vi "Launch Controller.vi"(8 "error in":errorcluster) -> ()   [LabVIEW 2015]
doc: "This VI executes continuously carrying out the current operation and responding to updates or new operations. It will often contain the timing or control code that is difficult to place directly in TeleOp. This VI generally opens all sensors and motors and isolates the rest of the robot code from knowing how the operations are carried out."
uses:
  Launch Operations.ctl
  Launch Setpoints.ctl
  <vilib>/Rock Robotics/WPI/SafetyOutput/WPI_SafetyOutputConfigMenu.ctl
  <vilib>/Rock Robotics/SystemInterfaces/DIO/FPGA_DIOPWMChannel.ctl
  <vilib>/addons/control/pid/NI_PID_pid.lvlib
  <vilib>/addons/control/pid/pid.llb/PID (DBL).vi
  <vilib>/Rock Robotics/WPI/MotorControl/WPI_MotorControlOpen SPARK.vi
  <vilib>/Rock Robotics/Network Tables/NT Write Boolean.vi
panel:
  in  "PID gains (flywheel R speed)":T1={"proportional gain (Kc)"=0.6, "integral time (Ti, min)"=0.01, "derivative time (Td, min)"=0.0}
  in  "Angle Tolerance":dbl=0.05 format="%#_13g"
  in  "PID gains (launcher angle set)":T1={"proportional gain (Kc)"=0.6, "integral time (Ti, min)"=0.01, "derivative time (Td, min)"=0.0}
  in  "PID gains (flywheel L speed)":T1={"proportional gain (Kc)"=0.6, "integral time (Ti, min)"=0.01, "derivative time (Td, min)"=0.0}
  out "Current\nCmd":string
  # "Tip: It may be helpful to observe inputs and sensor values.\nYou may also want to display tuning or debugging controls."
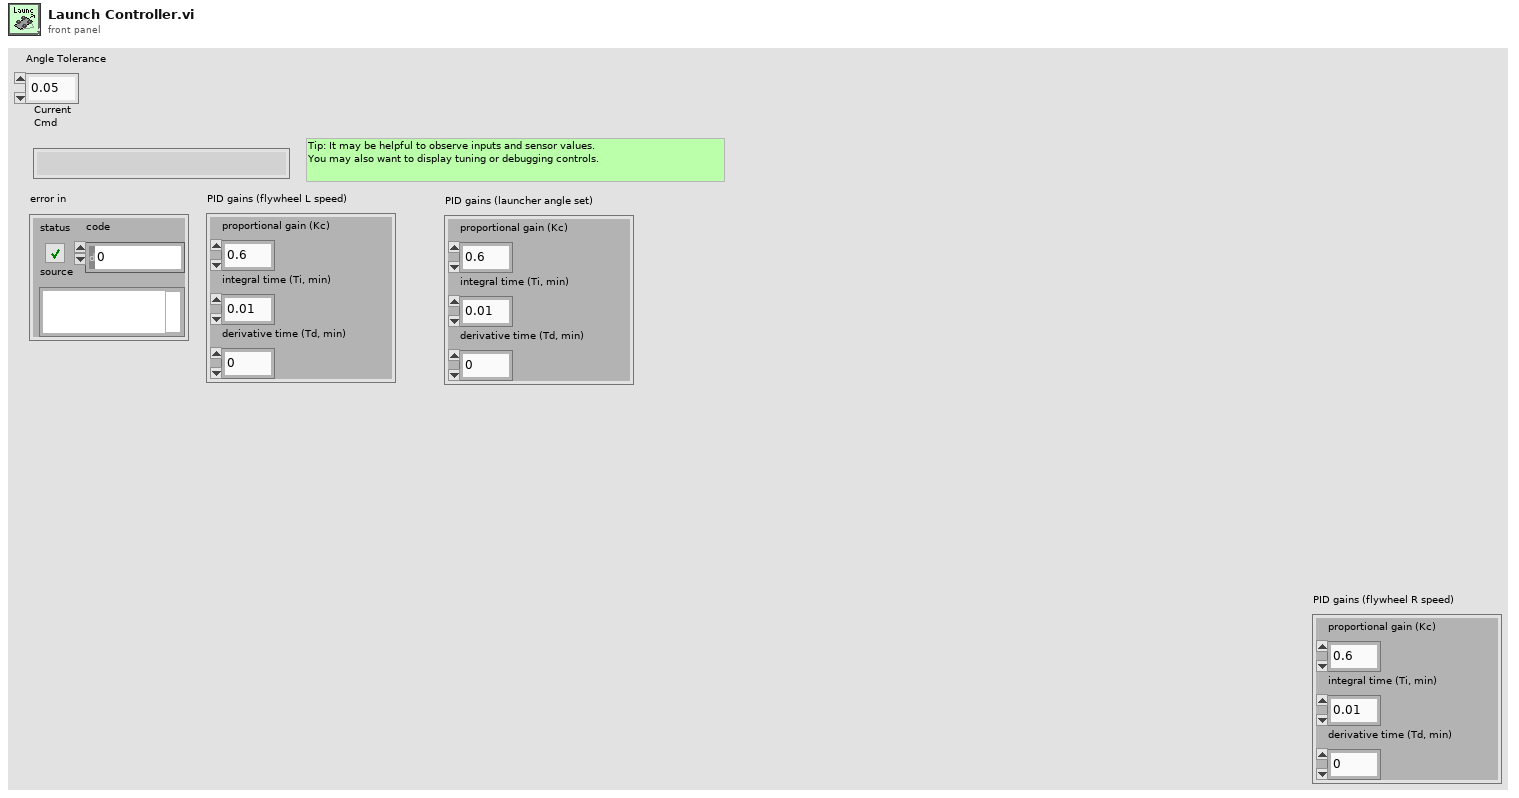
[diagram p1: front panel]
types:
  T1 = cluster{"proportional gain (Kc)":dbl, "integral time (Ti, min)":dbl, "derivative time (Td, min)":dbl}
  T2 = typedef "WPI_SafetyOutputConfigMenu.ctl" = enum16{"Enable", "Disable"}
  T3 = typedef "FPGA_DIOPWMChannel.ctl" = enum8{"PWM 0", "PWM 1", "PWM 2", "PWM 3", "PWM 4", "PWM 5", "PWM 6", "PWM 7", "PWM 8", "PWM 9", "PWM MXP 0", "PWM MXP 1", "PWM MXP 2", "PWM MXP 3", "PWM MXP 4", "PWM MXP 5", "PWM MXP 6", "PWM MXP 7", "PWM MXP 8", "PWM MXP 9", "Invalid"}
  T4 = typedef "Launch Setpoints.ctl" = cluster{"Operation":T5, "Setpoint":dbl, "Duration":dbl}
  T5 = typedef "Launch Operations.ctl" = enum16{"Reserve", "Read Current", "Immediate", "Zero", "Launcher Test", "Set Velocity", "Set Angle", "Manual Angle Test"}
  T6 = typedef "WPI_MotorControlDeviceRef.ctl" = cluster{"DeviceStatus":errorcluster, "Type":T7, "PWM":cluster{"PWM Channel":T3, "DeadBand":T8}, "CAN":cluster{"Device Number":u8, "Control Mode":T9, "Semaphore":T10, "Max Vout":dbl, "TalonSRX Control Mode":T11}, "Invert":bool}
  T7 = typedef "WPI_MotorControlType.ctl" = enum16{"PWM", "CAN", "CANTalonSRX"}
  T8 = typedef "WPI_PWMDeadband.ctl" = cluster{"Name":string, "maxPositivePwm":i32, "minPositivePwm":i32, "centerPwm":i32, "maxNegativePwm":i32, "minNegativePwm":i32, "angularRange":u16}
  T9 = typedef "WPI_CANJaguar_ControlMode.ctl" = enum8{"Percent VBus", "Current", "Speed", "Position", "Voltage"}
  T10 = typedef "Semaphore RefNum" = refnum<k1>
  T11 = typedef "WPI_CANTalonSRX_APIControlMode.ctl" = enum8{"Percent VBus", "Speed", "Position", "Slave", "Unchanged / Invalid", "Voltage Compensation", "Current", "Motion Profile"}
  T12 = typedef "WPI_SwitchDevRef.ctl" = cluster{"DevStatus":errorcluster, "DIO Channel":T13, "CntIndex":T14, "Normally Closed":bool}
  T13 = typedef "FPGA_DIOChannel.ctl" = enum8{"DIO 0", "DIO 1", "DIO 2", "DIO 3", "DIO 4", "DIO 5", "DIO 6", "DIO 7", "DIO 8", "DIO 9", "DIO MXP 0", "DIO MXP 1", "DIO MXP 2", "DIO MXP 3", "DIO MXP 4", "DIO MXP 5", "DIO MXP 6", "DIO MXP 7", "DIO MXP 8", "DIO MXP 9", "DIO MXP 10", "DIO MXP 11", "DIO MXP 12", "DIO MXP 13", "DIO MXP 14", "DIO MXP 15", "Invalid"}
  T14 = typedef "FPGA_CounterCtrSystemIndex.ctl" = enum8{"Ctr 0", "Ctr 1", "Ctr 2", "Ctr 3", "Ctr 4", "Ctr 5", "Ctr 6", "Ctr 7", "Invalid"}
  T15 = typedef "WPI_EncoderDevRef.ctl" = cluster{"DevStatus":errorcluster, "EncoderIndex":T16, "CounterIndex":T14, "DistancePerCount":dbl, "Decoding Type":T17}
  T16 = typedef "FPGA_EncoderIdx.ctl" = enum8{"Enc 0", "Enc 1", "Enc 2", "Enc 3", "Enc 4", "Enc 5", "Enc 6", "Enc 7", "Invalid"}
  T17 = typedef "WPI_EncoderType.ctl" = enum16{"1x", "2x", "4x"}
  T18 = typedef "Command Status Info.ctl" = cluster{"Name":string, "Status":T19, "notifier out":T20}
  T19 = typedef "Completion Status.ctl" = enum16{"Successful", "Aborted", "Incomplete"}
  T20 = typedef "Completion Notifier.ctl" = refnum<notifier>
  T21 = cluster{"Default Command":T4, "Command Timing":cluster{"Start Time (ms)":u32, "Iterations":i32}, "Command Arguments":cluster{"Command Info":T18, "Description":string, "Default Command":T4, "notifier out":refnum<notifier>, "Subsystem Name":string}}
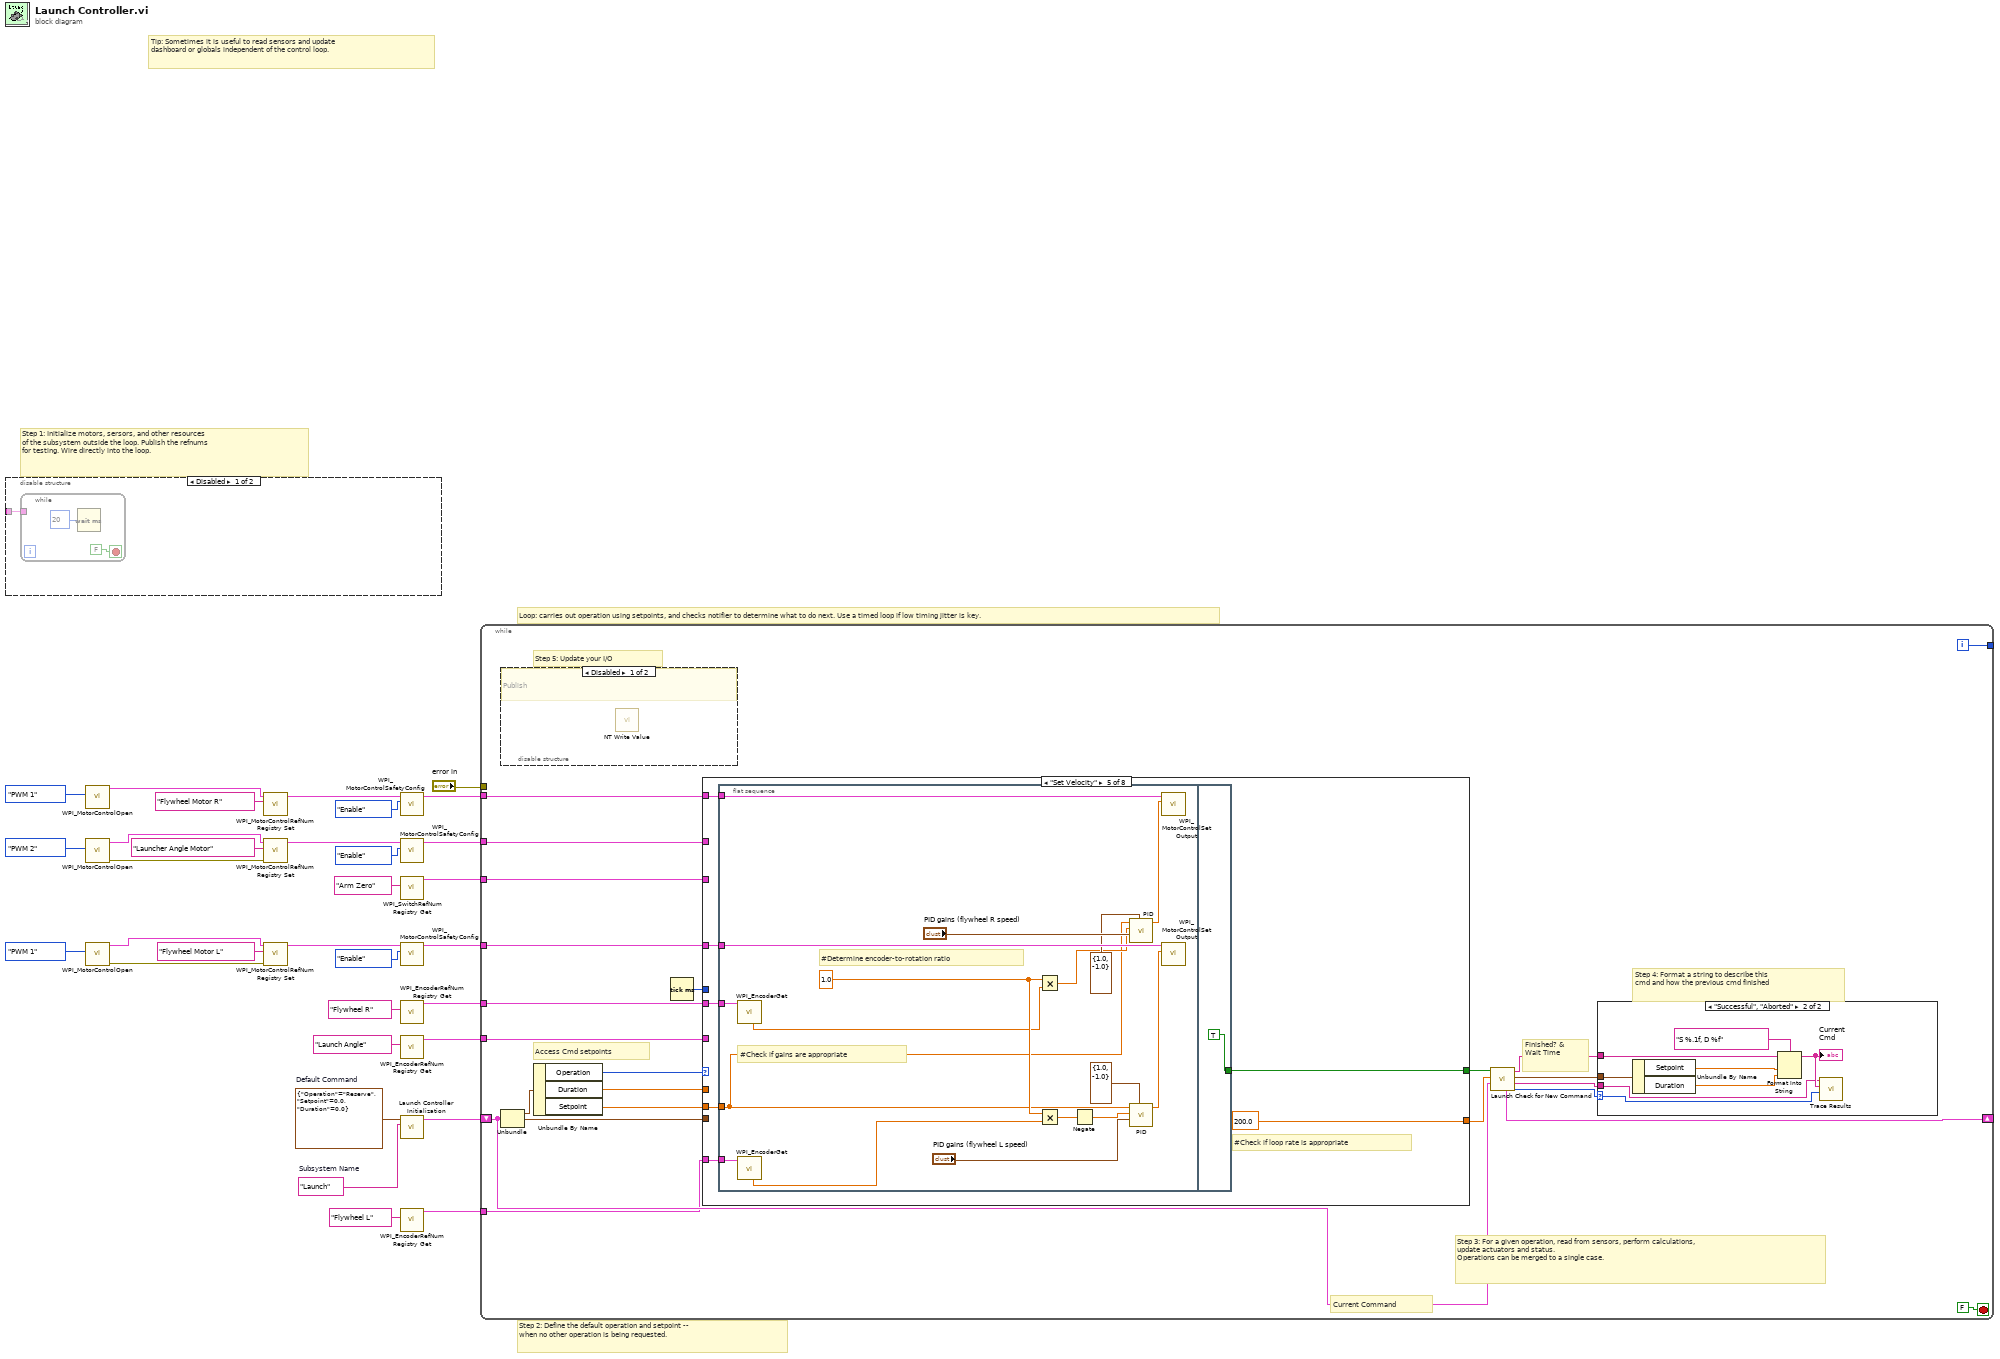
[diagram p0: block diagram]
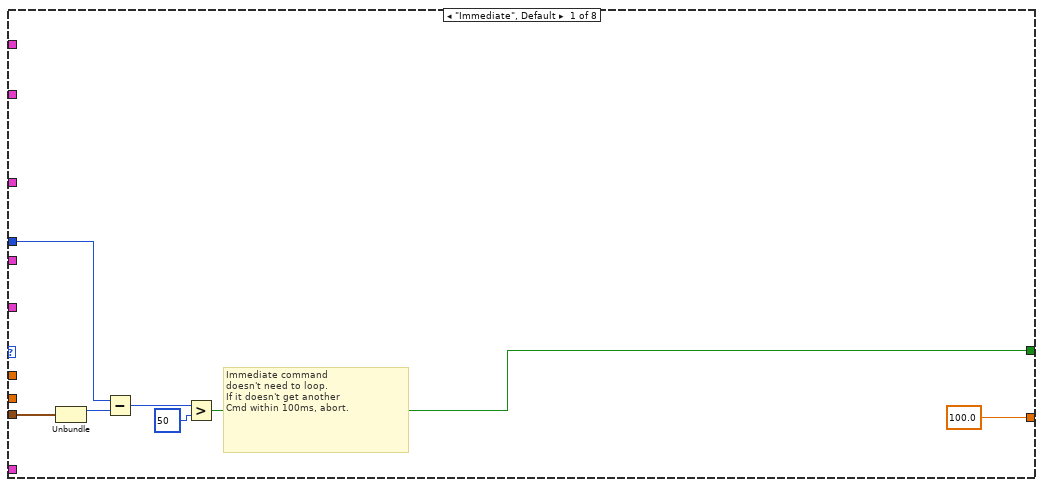
[diagram p5: hidden frame]
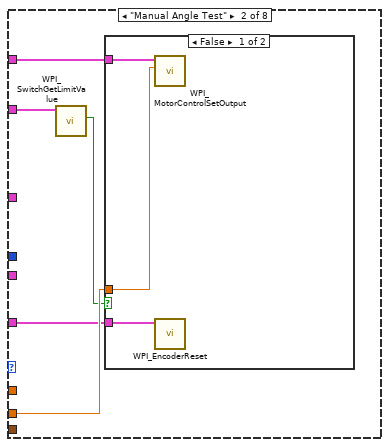
[diagram p6: hidden frame]
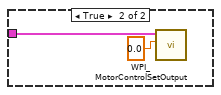
[diagram p7: hidden frame]
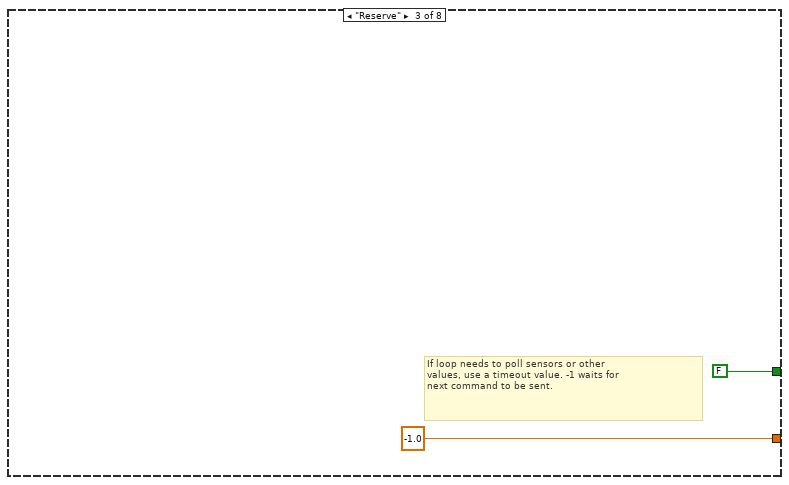
[diagram p8: hidden frame]
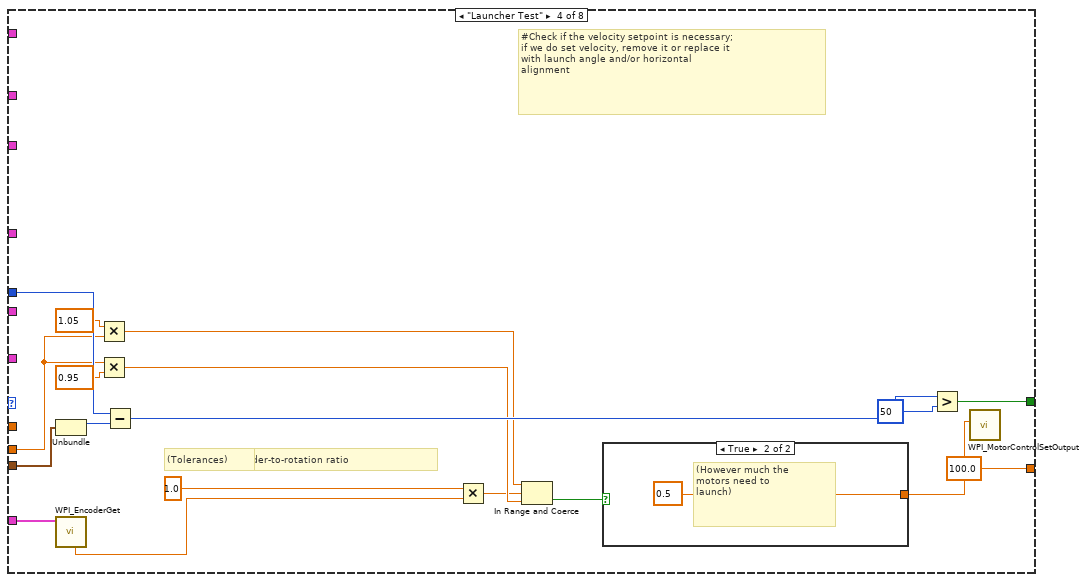
[diagram p9: hidden frame]
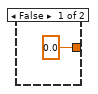
[diagram p10: hidden frame]
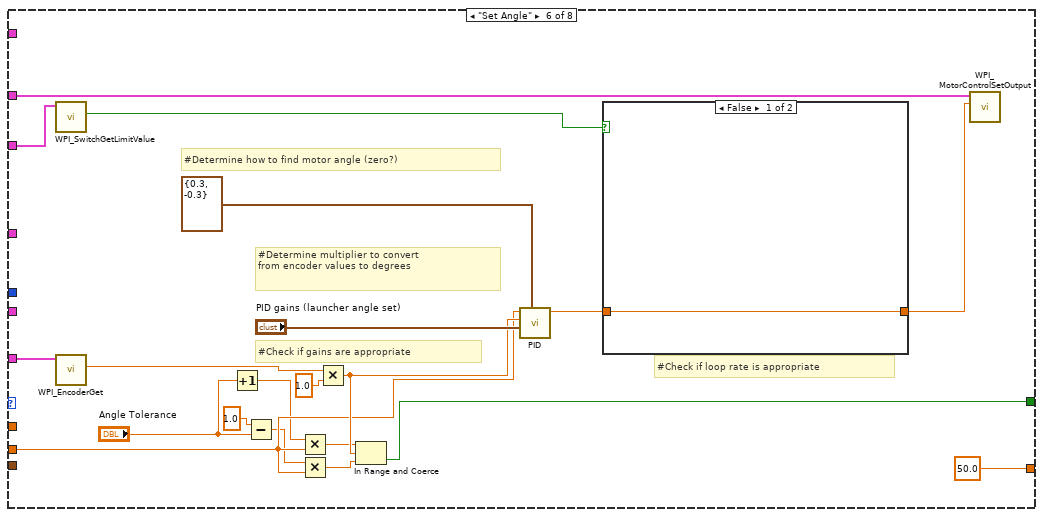
[diagram p11: hidden frame]
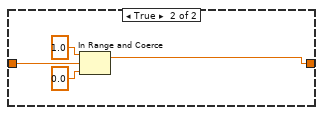
[diagram p12: hidden frame]
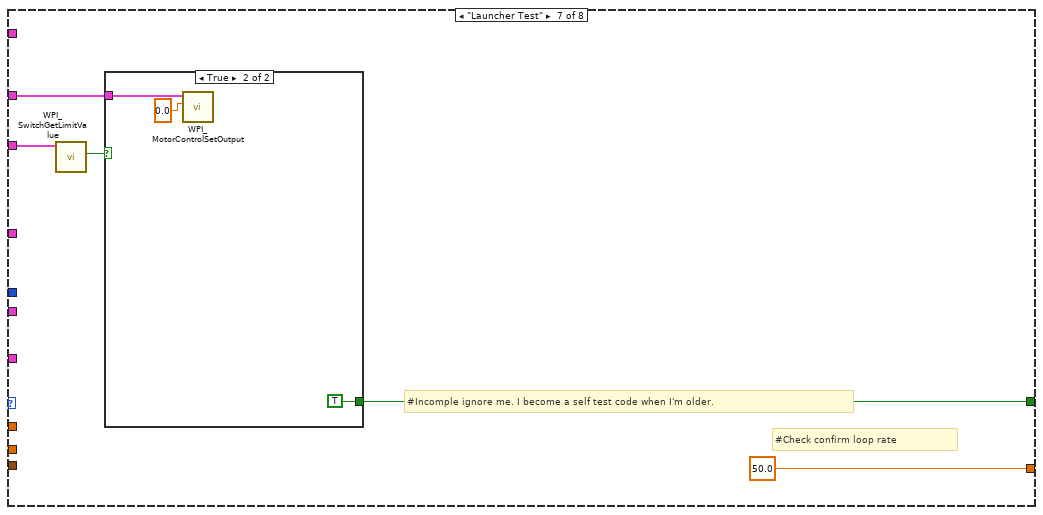
[diagram p13: hidden frame]
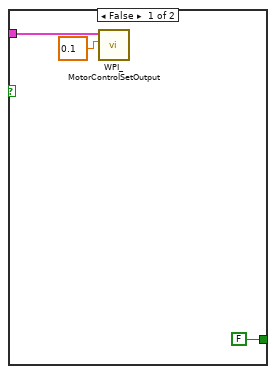
[diagram p14: hidden frame]
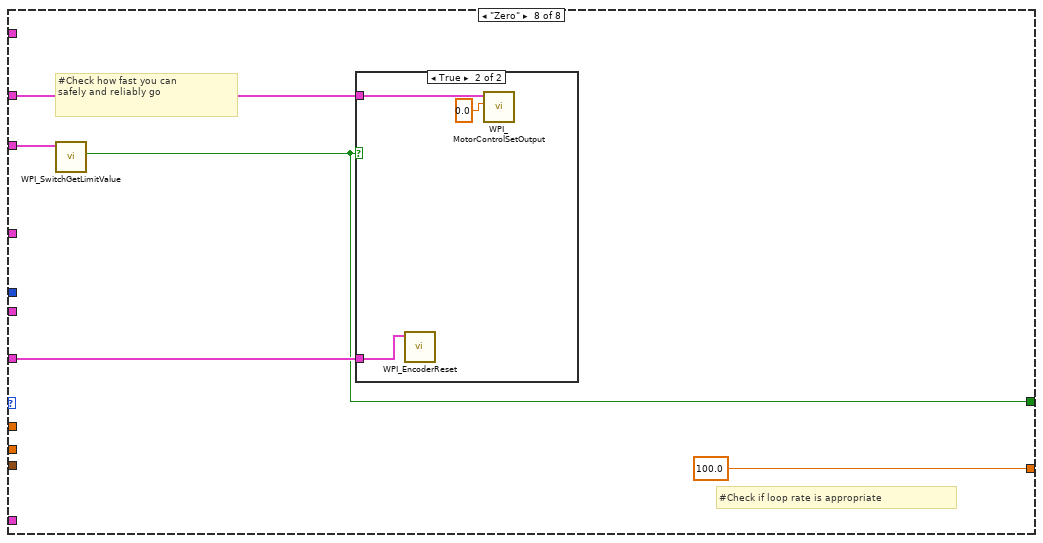
[diagram p15: hidden frame]
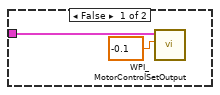
[diagram p16: hidden frame]
diagram:
  w29 = T4 {"Operation"=enum."Reserve", "Setpoint"=0.0, "Duration"=0.0}  # Default Command
  w30 = "Launch"  # Subsystem Name
  # "Tip: Sometimes it is useful to read sensors and update\ndashboard or globals independent of the control loop."
  # "Step 2: Define the default operation and setpoint --\nwhen no other operation is being requested."
  # "Step 1: Initialize motors, sersors, and other resources\nof the subsystem outside the loop. Publish the refnums\nfor testing. Wire directly into the loop."
  # "Loop: carries out operation using setpoints, and checks notifier to determine what to do next. Use a timed loop if low timing jitter is key."
  n1 = disable-structure shown="Disabled" {
    disable-tunnel: _ -> [w33 _]
    frame Disabled {
      n2 = while {
        tunnel: w33 -> [_]
        stop <- FALSE stop-if-true
        n3 = Wait (ms)(milliseconds to wait=u32 20) -> ()  [unwired: 1 out]
      }
    }
    frame Enabled {
    }
  }
  n4 = call-poly <vilib>:"WPI_MotorControlOpen.vi"("PWM Channel"=FPGA_DIOPWMChannel."PWM 1") -> ("MotorControlDeviceRef"=w4:T6)  [unwired: 9 in, 1 out]
  n5 = call-poly <vilib>:"WPI_MotorControlOpen.vi"("PWM Channel"=FPGA_DIOPWMChannel."PWM 2") -> ("error out"=w18:errorcluster, "MotorControlDeviceRef"=w20:T6)  [unwired: 9 in]
  n6 = call-poly <vilib>:"WPI_MotorControlOpen.vi"("PWM Channel"=FPGA_DIOPWMChannel."PWM 1") -> ("error out"=w25:errorcluster, "MotorControlDeviceRef"=w27:T6)  [unwired: 9 in]
  n7 = call <vilib>:"WPI_MotorControlRefNum Registry Set.vi"("refnum name"="Flywheel Motor R", "MotorControlDevRef"=w4) -> ("MotorControlDevRef"=w7:T6)  [unwired: 8 in, 1 out]
  n8 = call <vilib>:"WPI_MotorControlRefNum Registry Set.vi"("error in (no error)"=w18, "refnum name"="Launcher Angle Motor", "MotorControlDevRef"=w20) -> ("MotorControlDevRef"=w19:T6)  [unwired: 7 in, 1 out]
  n9 = call <vilib>:"WPI_MotorControlRefNum Registry Set.vi"("error in (no error)"=w25, "refnum name"="Flywheel Motor L", "MotorControlDevRef"=w27) -> ("MotorControlDevRef"=w26:T6)  [unwired: 7 in, 1 out]
  n10 = call <vilib>:"WPI_MotorControlSafetyConfig.vi"("mode"=WPI_SafetyOutputConfigMenu."Enable", "MotorControlDevRef"=w7) -> ("MotorControlDevRef"=w3:T6)  [unwired: 8 in, 1 out]
  n11 = call <vilib>:"WPI_MotorControlSafetyConfig.vi"("mode"=WPI_SafetyOutputConfigMenu."Enable", "MotorControlDevRef"=w19) -> ("MotorControlDevRef"=w15:T6)  [unwired: 8 in, 1 out]
  n12 = call <vilib>:"WPI_SwitchRefNum Registry Get.vi"("refnum name"="Arm Zero") -> ("SwitchDevRef"=w9:T12)  [unwired: 9 in, 1 out]
  n13 = call <vilib>:"WPI_MotorControlSafetyConfig.vi"("mode"=WPI_SafetyOutputConfigMenu."Enable", "MotorControlDevRef"=w26) -> ("MotorControlDevRef"=w22:T6)  [unwired: 8 in, 1 out]
  n14 = call <vilib>:"WPI_EncoderRefNum Registry Get.vi"("refnum name"="Flywheel R") -> ("EncoderDevRef"=w1:T15)  [unwired: 9 in, 1 out]
  n15 = call <vilib>:"WPI_EncoderRefNum Registry Get.vi"("refnum name"="Launch Angle") -> ("EncoderDevRef"=w13:T15)  [unwired: 9 in, 1 out]
  n16 = call "Launch Controller Initialization.vi"("Subsystem Name"=w30, "Default Command"=w29) -> ("Command Info"=w31:T21)  [unwired: 9 in]
  n17 = call <vilib>:"WPI_EncoderRefNum Registry Get.vi"("refnum name"="Flywheel L") -> ("EncoderDevRef"=w14:T15)  [unwired: 9 in, 1 out]
  n18 = while {
    shift-right: [w49] -> _
    shift-left: w31 -> [w50]
    tunnel: [w57] -> _
    tunnel: "error in" -> [_]
    tunnel: w22 -> [w39]
    tunnel: w14 -> [w42]
    tunnel: w15 -> [w40]
    tunnel: w13 -> [w41]
    tunnel: w9 -> [w38]
    tunnel: w3 -> [w36]
    tunnel: w1 -> [w37]
    i -> [w57]
    stop <- FALSE stop-if-true
    # "Step 5: Update your I/O"
    # "Step 4: Format a string to describe this\ncmd and how the previous cmd finished"
    # "Current Command"
    # "Access Cmd setpoints"
    # "Finished? &\nWait Time"
    # "Step 3: For a given operation, read from sensors, perform calculations,\nupdate actuators and status.\nOperations can be merged to a single case."
    n19 = disable-structure shown="Disabled" {
      frame Disabled {
        # "Publish"
        n20 = call-poly <vilib>:"NT Write Value.vi"() -> ()  [unwired: 11 in, 1 out]
      }
      frame Enabled {
      }
    }
    n21 = Unbundle(w50) -> ("Default Command"=w56:T4, "Command Timing"=w52:cluster{"Start Time (ms)":u32, "Iterations":i32})  [unwired: 1 out]
    n22 = Unbundle By Name(w56) -> ("Operation"=w55:T5, "Duration"=w54:dbl, "Setpoint"=w51:dbl)
    n23 = Tick Count (ms)() -> (millisecond timer value=w53:u32)
    n24 = case shown="\"Set Velocity\"" w55 {
      tunnel: [100.0 _ -1.0 100.0 200.0 50.0 50.0 100.0] -> w47
      tunnel: [w67 _ FALSE ("ignore previous (F)") w98 w106 w139 w158 w167] -> w48
      tunnel: w52 -> [w69 _ _ w100 _ _ _ _]
      tunnel: w54 -> [_ _ _ _ _ _ _ _]
      tunnel: w53 -> [w68 _ _ w99 _ _ _ _]
      tunnel: w51 -> [_ w78 _ w90 w108 w142 _ _]
      tunnel: w42 -> [_ _ _ w91 w112 _ _ _]
      tunnel: w41 -> [_ w74 _ _ _ w148 _ w169]
      tunnel: w40 -> [_ w77 _ _ _ w144 w156 w170]
      tunnel: w39 -> [_ _ _ _ w110 _ _ _]
      tunnel: w38 -> [_ w76 _ _ _ w134 w160 w171]
      tunnel: w37 -> [_ _ _ _ w109 _ _ _]
      tunnel: w36 -> [_ _ _ _ w107 _ _ _]
      frame "Immediate", Default {
        # "Immediate command\ndoesn't need to loop.\nIf it doesn't get another\nCmd within 100ms, abort."
        n25 = Unbundle(w69) -> ("Start Time (ms)"=w72:u32)  [unwired: 1 out]
        n26 = Subtract(x=w68, y=w72) -> (x-y=w71:u32)
        n27 = Greater?(x=w71, y=u8 50 ("Left Motor")) -> (0:w67:bool)
      }
      frame "Manual Angle Test" {
        n28 = call <vilib>:"WPI_SwitchGetLimitValue.vi"("SwitchDevRef"=w76) -> ("Switch Pressed"=w75:bool)  [unwired: 8 in, 2 out]
        n29 = case shown="False" w75 {
          tunnel: w78 -> [w81 _]
          tunnel: w77 -> [w80 w82]
          tunnel: w74 -> [w79 _]
          frame False {
            n30 = call <vilib>:"WPI_MotorControlSetOutput.vi"("Output"=w81, "MotorControlDevRef"=w80) -> ()  [unwired: 7 in, 3 out]
            n31 = call <vilib>:"WPI_EncoderReset.vi"("EncoderDevRef"=w79) -> ()  [unwired: 9 in, 2 out]
          }
          frame True {
            n32 = call <vilib>:"WPI_MotorControlSetOutput.vi"("Output"=0.0, "MotorControlDevRef"=w82) -> ()  [unwired: 7 in, 3 out]
          }
        }
      }
      frame "Reserve" {
        # "If loop needs to poll sensors or other\nvalues, use a timeout value. -1 waits for\nnext command to be sent."
      }
      frame "Launcher Test" {
        # "#Check if the velocity setpoint is necessary;\nif we do set velocity, remove it or replace it\nwith launch angle and/or horizontal\nalignment"
        # "#Determine encoder-to-rotation ratio"
        # "(Tolerances)"
        n33 = Unbundle(w100) -> ("Start Time (ms)"=w101:u32)  [unwired: 1 out]
        n34 = call <vilib>:"WPI_EncoderGet.vi"("EncoderDevRef"=w91) -> ("Rate"=w87:dbl)  [unwired: 5 in, 5 out]
        n35 = Multiply(x=1.05, y=w90) -> (x*y=w95:dbl)
        n36 = Multiply(x=w90, y=0.95) -> (x*y=w94:dbl)
        n37 = Subtract(x=w99, y=w101) -> (x-y=w102:u32)
        n38 = Multiply(x=1.0, y=w87) -> (x*y=w86:dbl)
        n39 = In Range and Coerce(upper limit=w95, x=w86, lower limit=w94) -> (In Range?=w96:bool)  [unwired: 1 out]
        n40 = case shown="True" w96 {
          tunnel: [0.0 0.5] -> w89
          frame False {
          }
          frame True {
            # "(However much the\nmotors need to\nlaunch)"
          }
        }
        n41 = Greater?(x=w102, y=u8 50 ("Left Motor")) -> (0:w98:bool)
        n42 = call <vilib>:"WPI_MotorControlSetOutput.vi"("Output"=w89) -> ()  [unwired: 8 in, 3 out]
      }
      frame "Set Velocity" {
        # "#Check if loop rate is appropriate"
        n43 = flat-sequence {
          tunnel: w112 -> [w129]
          tunnel: w110 -> [w126]
          tunnel: w109 -> [w125]
          tunnel: w108 -> [w117]
          tunnel: w107 -> [w114]
          tunnel: [TRUE] -> w106
          frame #0 {
            w118 = 1.0
            # "#Determine encoder-to-rotation ratio"
            # "#Check if gains are appropriate"
            n44 = call <vilib>:"WPI_EncoderGet.vi"("EncoderDevRef"=w125) -> ("Rate"=w116:dbl)  [unwired: 5 in, 5 out]
            n45 = call <vilib>:"WPI_EncoderGet.vi"("EncoderDevRef"=w129) -> ("Rate"=w128:dbl)  [unwired: 5 in, 5 out]
            n46 = Multiply(x=w118, y=w116) -> (x*y=w119:dbl)
            n47 = Multiply(x=w118, y=w128) -> (x*y=w122:dbl)
            n48 = Negate(x=w122) -> (-x=w113:dbl)
            n49 = call-poly <vilib>:"PID.vi"("output range"=cluster{"output high":dbl, "output low":dbl} {"output high"=1.0, "output low"=-1.0}, "PID gains"="PID gains (flywheel R speed)", "process variable"=w119, "setpoint"=w117) -> ("output"=w115:dbl)  [unwired: 6 in, 1 out]
            n50 = call-poly <vilib>:"PID.vi"("output range"=cluster{"output high":dbl, "output low":dbl} {"output high"=1.0, "output low"=-1.0}, "PID gains"="PID gains (flywheel L speed)", "process variable"=w113, "setpoint"=w117) -> ("output"=w127:dbl)  [unwired: 6 in, 1 out]
            n51 = call <vilib>:"WPI_MotorControlSetOutput.vi"("Output"=w115, "MotorControlDevRef"=w114) -> ()  [unwired: 7 in, 3 out]
            n52 = call <vilib>:"WPI_MotorControlSetOutput.vi"("Output"=w127, "MotorControlDevRef"=w126) -> ()  [unwired: 7 in, 3 out]
          }
          frame #1 {
          }
        }
      }
      frame "Set Angle" {
        # "#Determine multiplier to convert \nfrom encoder values to degrees"
        # "#Check if loop rate is appropriate"
        # "#Determine how to find motor angle (zero?)"
        # "#Check if gains are appropriate"
        n53 = call <vilib>:"WPI_SwitchGetLimitValue.vi"("SwitchDevRef"=w134) -> ("Switch Pressed"=w133:bool)  [unwired: 8 in, 2 out]
        n54 = call <vilib>:"WPI_EncoderGet.vi"("EncoderDevRef"=w148) -> ("Distance"=w146:dbl)  [unwired: 5 in, 5 out]
        n55 = Increment(x="Angle Tolerance") -> (x+1=w138:dbl)
        n56 = Subtract(x=1.0, y="Angle Tolerance") -> (x-y=w135:dbl)
        n57 = Multiply(x=w138, y=w142) -> (x*y=w141:dbl)
        n58 = Multiply(x=w135, y=w142) -> (x*y=w140:dbl)
        n59 = Multiply(x=w146, y=1.0) -> (x*y=w143:dbl)
        n60 = In Range and Coerce(upper limit=w141, x=w143, lower limit=w140) -> (In Range?=w139:bool)  [unwired: 1 out]
        n61 = call-poly <vilib>:"PID.vi"("output range"=cluster{"output high":dbl, "output low":dbl} {"output high"=0.3, "output low"=-0.3}, "PID gains"="PID gains (launcher angle set)", "process variable"=w143, "setpoint"=w142) -> ("output"=w132:dbl)  [unwired: 6 in, 1 out]
        n62 = case shown="False" w133 {
          tunnel: w132 -> [w151 w155]
          tunnel: [w151 w152] -> w131
          frame False {
          }
          frame True {
            n63 = In Range and Coerce(upper limit=1.0, x=w155, lower limit=0.0) -> (coerced(x)=w152:dbl)  [unwired: 1 out]
          }
        }
        n64 = call <vilib>:"WPI_MotorControlSetOutput.vi"("Output"=w131, "MotorControlDevRef"=w144) -> ()  [unwired: 7 in, 3 out]
      }
      frame "Launcher Test" {
        # "#Incomple ignore me. I become a self test code when I'm older."
        # "#Check confirm loop rate"
        n65 = call <vilib>:"WPI_SwitchGetLimitValue.vi"("SwitchDevRef"=w160) -> ("Switch Pressed"=w159:bool)  [unwired: 8 in, 2 out]
        n66 = case shown="True" w159 {
          tunnel: [FALSE TRUE] -> w158
          tunnel: w156 -> [w162 w165]
          frame False {
            n67 = call <vilib>:"WPI_MotorControlSetOutput.vi"("Output"=0.1, "MotorControlDevRef"=w162) -> ()  [unwired: 7 in, 3 out]
          }
          frame True {
            n68 = call <vilib>:"WPI_MotorControlSetOutput.vi"("Output"=0.0, "MotorControlDevRef"=w165) -> ()  [unwired: 7 in, 3 out]
          }
        }
      }
      frame "Zero" {
        # "#Check if loop rate is appropriate"
        # "#Check how fast you can\nsafely and reliably go"
        n69 = call <vilib>:"WPI_SwitchGetLimitValue.vi"("SwitchDevRef"=w171) -> ("Switch Pressed"=w167:bool)  [unwired: 8 in, 2 out]
        n70 = case shown="True" w167 {
          tunnel: w170 -> [w172 w175]
          tunnel: w169 -> [_ w176]
          frame False {
            n71 = call <vilib>:"WPI_MotorControlSetOutput.vi"("Output"=-0.1, "MotorControlDevRef"=w172) -> ()  [unwired: 7 in, 3 out]
          }
          frame True {
            n72 = call <vilib>:"WPI_EncoderReset.vi"("EncoderDevRef"=w176) -> ()  [unwired: 9 in, 2 out]
            n73 = call <vilib>:"WPI_MotorControlSetOutput.vi"("Output"=0.0, "MotorControlDevRef"=w175) -> ()  [unwired: 7 in, 3 out]
          }
        }
      }
    }
    n74 = call "Launch Check for New Command.vi"("Current Command"=w50, "Wait time (ms)"=w47, "Finished?"=w48) -> ("Completion"=w43:T19, "Subsystem Name"=w44:string, "Current Command"=w45:T4, "Initial Trace String"=w46:string, "NextCommand"=w49:T21)  [unwired: 4 in]
    n75 = case shown="\"Successful\", \"Aborted\"" w43 {
      selector: w43 -> [_ w66]
      tunnel: w46 -> [_ w62]
      tunnel: w45 -> [_ w63]
      tunnel: w44 -> [_ w59]
      frame "Incomplete", Default {
        # "Continuing current command"
      }
      frame "Successful", "Aborted" {
        # "Report and setup for next command"
        n76 = Unbundle By Name(w63) -> ("Setpoint"=w65:dbl, "Duration"=w60:dbl)
        n77 = Format Into String(format string="S %.1f, D %f", initial string=w62, w65, w60) -> (resulting string=w61:string)  [unwired: 1 in, 1 out]
        "Current\nCmd" <- w61
        n78 = call <vilib>:"Trace Results.vi"("Status of previous command"=w66, "Description"=w61, "Subsystem"=w59) -> ()  [unwired: 9 in]
      }
    }
  }
